vi "Locate and Display Breakdown.vi"(8 "error in (no error)":errorcluster, 9 "Microphone Locations":cluster{"r":dbl, "theta":dbl, "z":dbl}[](array[cluster]), 10 "Correlation Region (ms)":cluster{dbl, dbl}(slide)={0.9, 0.6} scale=0.0..2.0, 11 "Signals":waveform(dbl)[](array[waveform])) -> (0 "error out":errorcluster, 1 "Side View Scene":refnum<vi>, 2 "Downstream View Scene":refnum<vi>, 3 "Upstream View Scene":refnum<vi>, 4 "Coordinates (cm, rad, cm)":cluster{"r":sgl, "theta":sgl, "z":sgl}[](array[cluster]))   [LabVIEW 2013, in "Breakdown Acoustics Controls.lvlib"]
uses:
  Breakdown Acoustics Controls.lvlib
panel:
  in  "Sample Rate":i32=100000
  out "Processed Signals":waveform(dbl)[](graph)
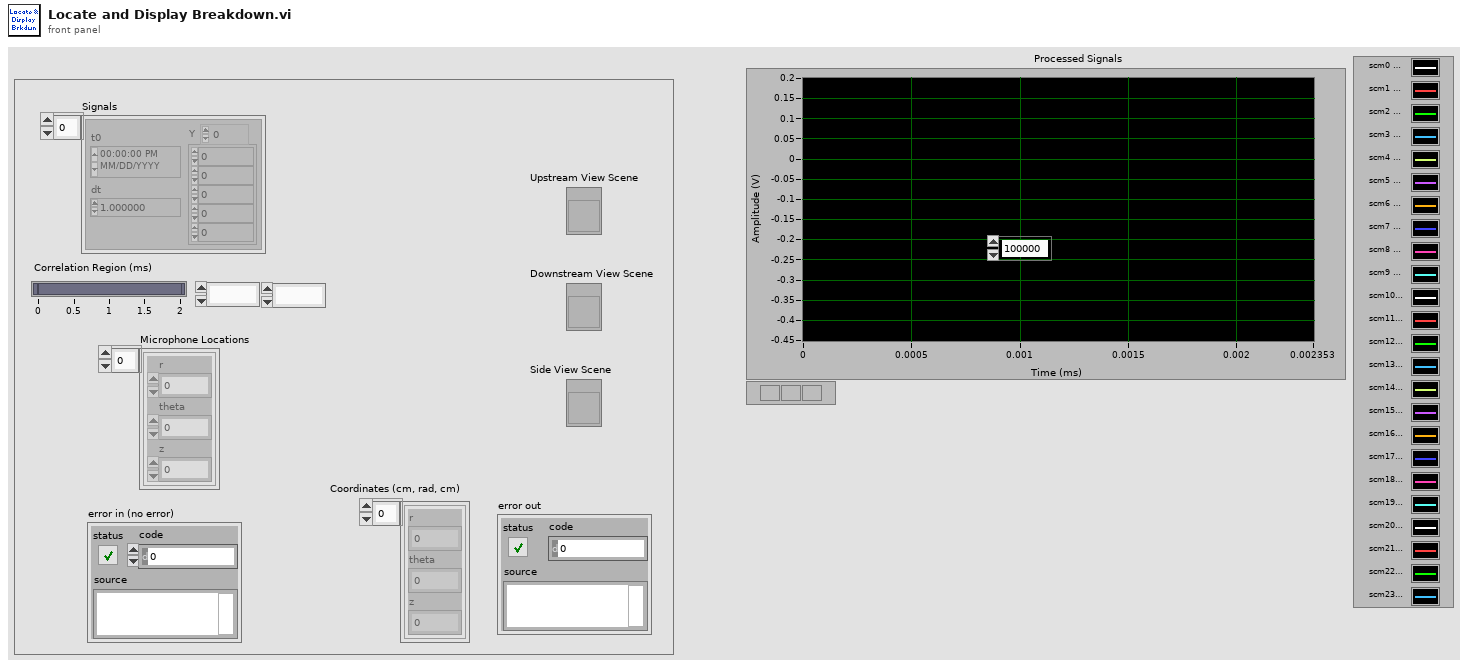
[diagram p1: front panel]
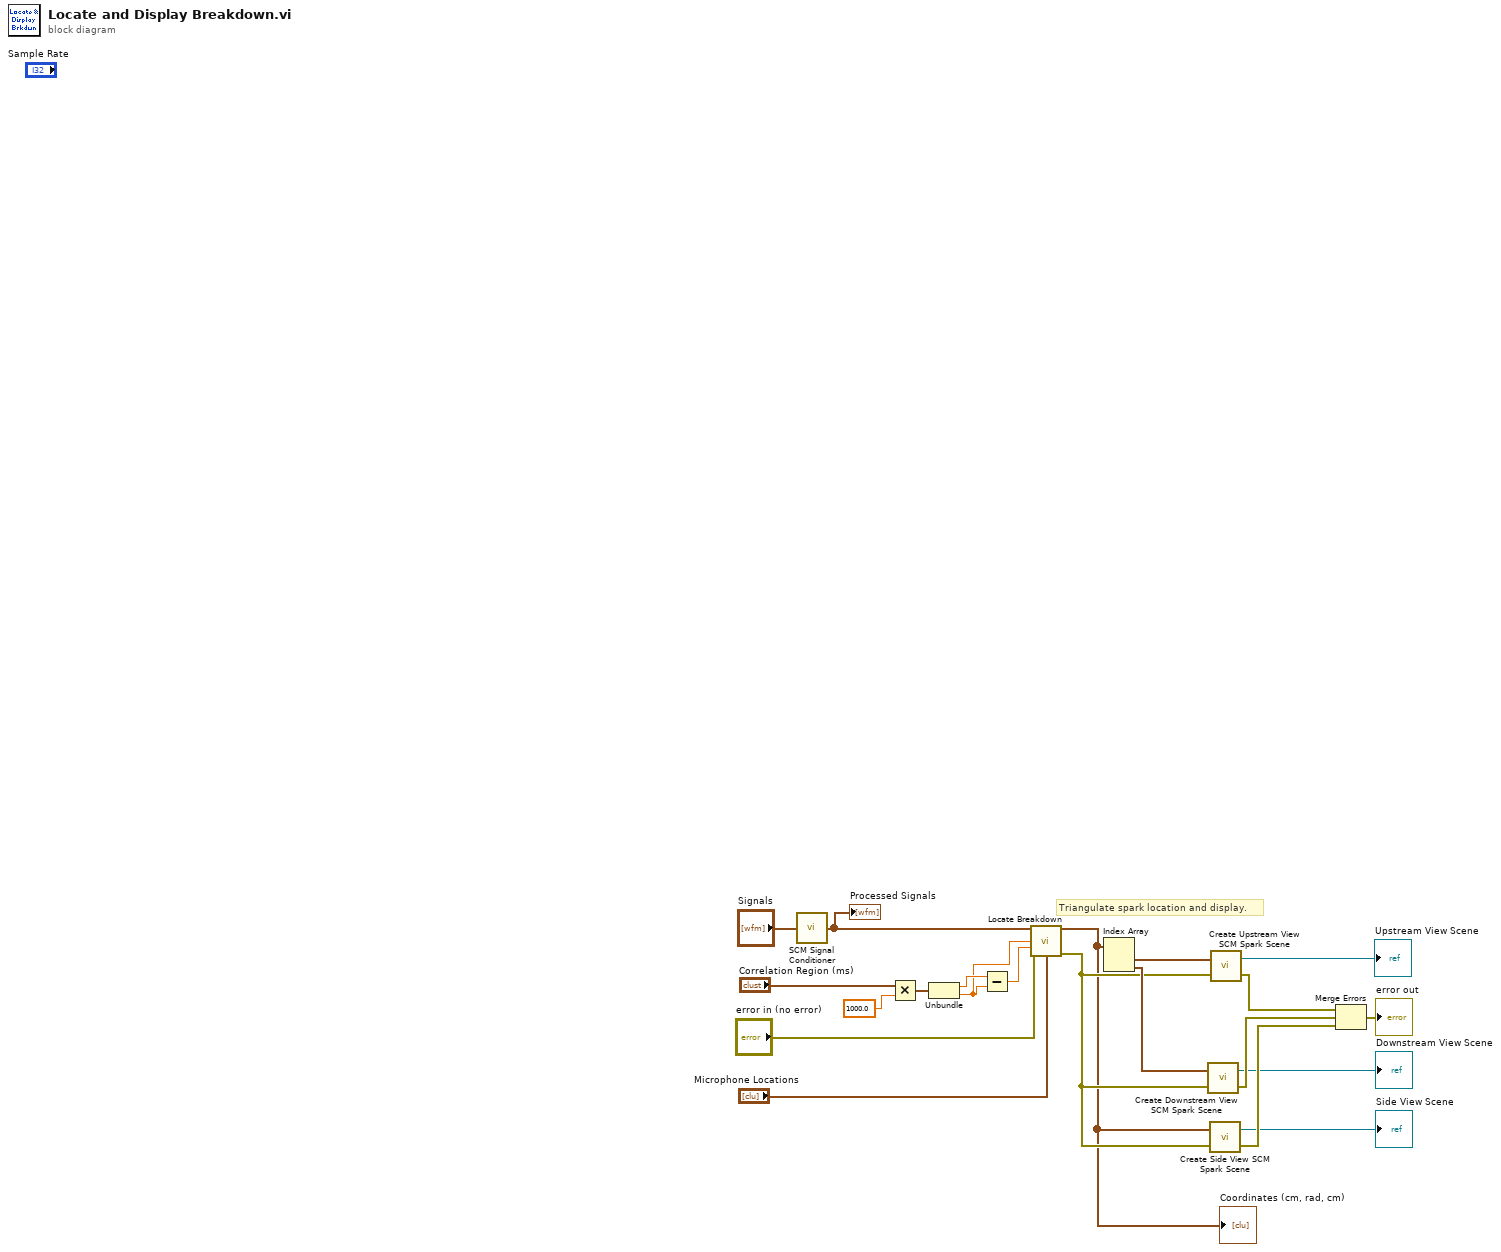
[diagram p0: block diagram]
diagram:
  # "Triangulate spark location and display."
  n1 = call "SCM Signal Conditioner.vi"("Signals"="Signals") -> ("Conditioned Signals"=w8:waveform(dbl)[])  [unwired: 4 in]
  "Processed Signals" <- w8
  n2 = Multiply(x="Correlation Region (ms)", y=1000.0) -> (x*y=w17:cluster{dbl, dbl})
  n3 = Unbundle(w17) -> (w16:dbl, w15:dbl)
  n4 = Subtract(x=w16, y=w15) -> (x-y=w14:dbl)
  n5 = call "Locate Breakdown.vi"("Signals"=w8, "Offset (µs)"=w15, "Duration (µs)"=w14, "error in (no error)"="error in (no error)", "Microphone Coordinates (cm, rad, cm)"="Microphone Locations") -> ("Coordinates (cm, rad, cm)"=w9:cluster{"r":sgl, "theta":sgl, "z":sgl}[], "error out"=w12:errorcluster)  [unwired: 8 in, 1 out]
  "Coordinates (cm, rad, cm)" <- w9
  n6 = Index Array(array=w9) -> (element #1=w20:cluster{"r":sgl, "theta":sgl, "z":sgl}, element #2=w13:cluster{"r":sgl, "theta":sgl, "z":sgl})  [unwired: 2 in]
  n7 = call "Create Downstream View SCM Spark Scene.vi"("error in (no error)"=w12, "Spark Coordinates (cm, rad, cm)"=w13) -> ("error out"=w11:errorcluster, "reference out"=→"Downstream View Scene":refnum<vi>)
  n8 = call "Create Side View SCM Spark Scene.vi"("error in (no error)"=w12, "Spark Coordinates (cm, rad, cm)"=w9) -> ("error out"=w10:errorcluster, "reference out"=→"Side View Scene":refnum<vi>)
  n9 = call "Create Upstream View SCM Spark Scene.vi"("error in (no error)"=w12, "Spark Coordinates (cm, rad, cm)"=w20) -> ("error out"=w21:errorcluster, "reference out"=→"Upstream View Scene":refnum<vi>)
  n10 = Merge Errors(w21, w11, w10) -> (→"error out":errorcluster)
